vi "Decode TempValue.vi"(8 "error in (no error)":errorcluster caption="错误输入（无错误）", 11 "PanelRootNode 输入":refnum<class "PanelRootNode.lvclass"> caption="DNL_LabVIEW Object in") -> (0 "error out":errorcluster caption="错误输出", 2 "TempValues":string[][](array[string]), 3 "PanelRootNode 输出":refnum<class "PanelRootNode.lvclass"> caption="DNL_LabVIEW Object out")   [LabVIEW 2016, in "PanelRootNode.lvclass"]
uses:
  PanelRootNode.lvclass
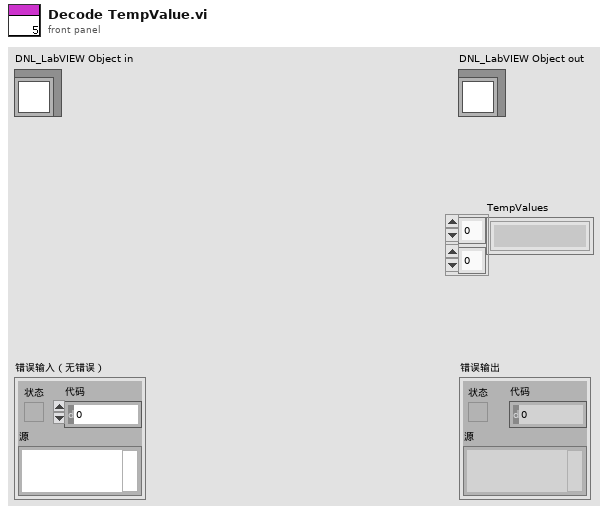
[diagram p1: front panel]
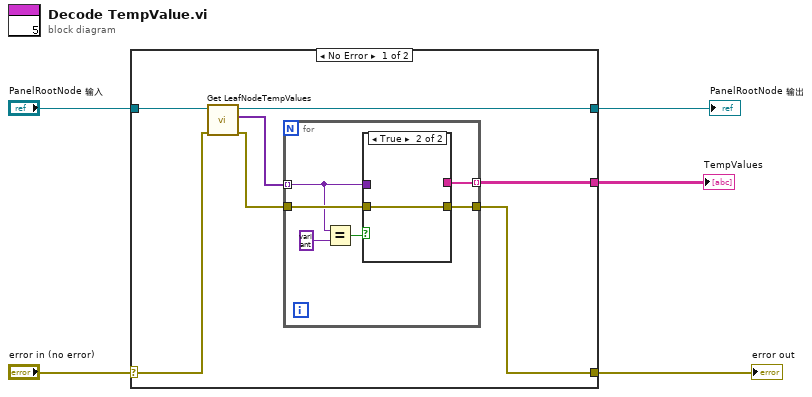
[diagram p0: block diagram]
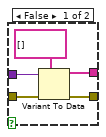
[diagram p2: hidden frame]
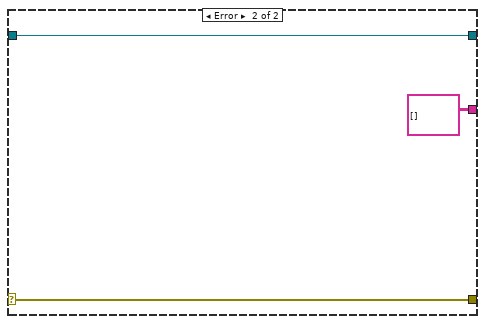
[diagram p3: hidden frame]
diagram:
  n1 = case shown="No Error" "error in (no error)" {
    selector: "error in (no error)" -> [w8 w27]
    tunnel: [w7 w27] -> w4
    tunnel: [w11 w26] -> w2
    tunnel: "PanelRootNode 输入" -> [w12 w26]
    tunnel: [w6 string[][] []] -> w1
    frame No Error {
      n2 = call "Get LeafNodeTempValues.vi"("error in (no error)"=w8, "PanelRootNode 输入"=w12) -> ("error out"=w9:errorcluster, "TempValue"=w10:variant[], "PanelRootNode 输出"=w11:refnum<class "PanelRootNode.lvclass">)  [unwired: 7 in]
      n3 = for {
        tunnel: w10 -> [w15] mode=indexing
        tunnel: [w18] -> w6 mode=indexing
        tunnel: w9 -> [w17]
        tunnel: [w16] -> w7
        n4 = Equal?(x=w15, y=variant) -> (x = y?=w13:bool)
        n5 = case shown="True" w13 {
          tunnel: [w22 _] -> w18
          tunnel: w17 -> [w21 w24]
          tunnel: [w20 w24] -> w16
          tunnel: w15 -> [w19 _]
          frame False {
            n6 = Variant To Data(error in=w21, type=string[] [], Variant=w19) -> (data=w22:string[], error out=w20:errorcluster)
          }
          frame True {
          }
        }
      }
    }
    frame Error {
    }
  }
  "error out" <- w4
  "PanelRootNode 输出" <- w2
  "TempValues" <- w1
